vi "pharosOpenDynReg.vi"   [LabVIEW 2017]
uses:
  <vilib>/DAQmx/write.llb/DAQmx Write (Digital 1D U8 1Chan NSamp).vi
  globalDevices.vi
  <vilib>/DAQmx/create/channels.llb/DAQmx Create Channel (DO-Digital Output).vi
  <vilib>/DAQmx/configure/timing.llb/DAQmx Timing (Sample Clock).vi
  <vilib>/DAQmx/miscellaneous.llb/DAQmx Fill In Error Info.vi
  <resource>/objmgr/daqmx.rc
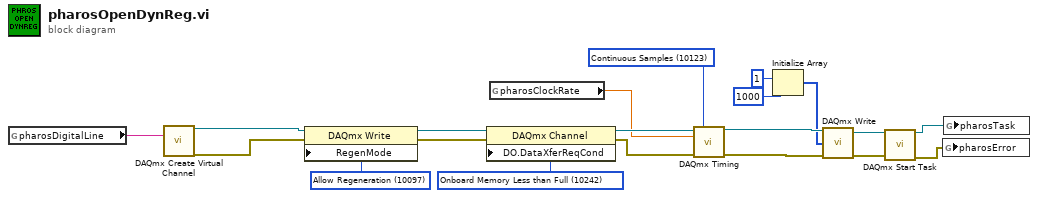
[diagram p0: block diagram]
diagram:
  w13 = 10123 items=["Finite Samples"=10178, "Continuous Samples"=10123, "Hardware Timed Single Point"=12522] ("sample mode")
  w17 = 10242 items=["Onboard Memory Empty"=10235, "Onboard Memory Half Full or Less"=10239, "Onboard Memory Less than Full"=10242] ("AO.DataXferReqCond")
  w20 = 10097 items=["Allow Regeneration"=10097, "Do Not Allow Regeneration"=10158] ("RegenMode")
  n1 = global read "globalDevices.vi" "pharosDigitalLine"() -> (w10:tag)
  n2 = call-poly <vilib>:"DAQmx Create Virtual Channel.vi"("lines"=w10) -> ("task out"=w12:refnum<k21>, "error out"=w11:errorcluster)  [unwired: 13 in]
  n3 = property class="DAQmx Write"(reference=w12, error in=w11, "RegenMode"=w20) -> (reference out=w19:refnum<k21>, error out=w18:errorcluster)
  n4 = property class="DAQmx Channel"(reference=w19, error in=w18, "DO.DataXferReqCond"=w17) -> (reference out=w16:refnum<k21>, error out=w15:errorcluster)
  n5 = global read "globalDevices.vi" "pharosClockRate"() -> (w14:dbl)
  n6 = call-poly <vilib>:"DAQmx Timing.vi"("task/channels in"=w16, "sample mode"=w13, "rate"=w14, "error in"=w15) -> ("task out"=w9:refnum<k21>, "error out"=w8:errorcluster)  [unwired: 10 in]
  n7 = Initialize Array(u8 1 ("element"), 1000 ("dimension size")) -> (w6:u8[])
  n8 = call-poly <vilib>:"DAQmx Write.vi"("task/channels in"=w9, "data"=w6, "error in"=w8) -> ("task out"=w4:refnum<k21>, "error out"=w3:errorcluster)  [unwired: 10 in, 1 out]
  n9 = call <vilib>:"DAQmx Start Task.vi"("task/channels in"=w4, "error in"=w3) -> ("task out"=w2:refnum<k21>, "error out"=w1:errorcluster)  [unwired: 12 in]
  n10 = global write "globalDevices.vi" "pharosError"(w1) -> ()
  n11 = global write "globalDevices.vi" "pharosTask"(w2) -> ()
